vi "gentec-M-Link.get Offset.vi"(1 "Offset DAC Code":i32) -> (0 "Offset [V]":dbl)   [LabVIEW 2014, in "gentec-M-Link - Driver.lvlib"]
doc: "This VI scales the DAC Code Offset (0 ... 4095) to the Offset in Volt (0 ... 2.5V)."
uses:
  gentec-M-Link - Driver.lvlib
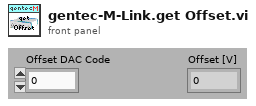
[diagram p1: front panel]
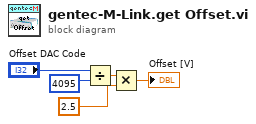
[diagram p0: block diagram]
diagram:
  n1 = Divide(x="Offset DAC Code", y=4095) -> (x/y=w3:dbl)
  n2 = Multiply(x=w3, y=2.5) -> (x*y=→"Offset [V]":dbl)
